vi "2nd_Derivative_Calc_Histogram.vi"(3 "[IN] delta":u16=1 min=1 max=50 step=1, 4 "[IN] Threshold value":u16, 5 "[IN] 1D Sorted Reversed Img":u16[](array[numeric])) -> (1 "[OUT] 2nd Derivative":dbl)   [LabVIEW 2020]
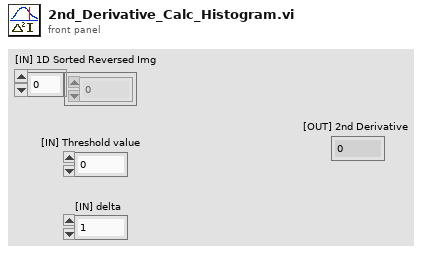
[diagram p1: front panel]
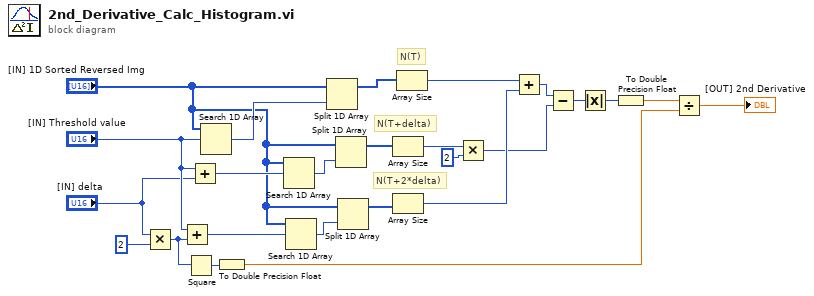
[diagram p0: block diagram]
diagram:
  # "N(T+2*delta)"
  # "N(T+delta)"
  # "N(T)"
  n1 = Multiply(x="[IN] delta", y=u16 2) -> (x*y=w15:u16)
  n2 = Add(x="[IN] Threshold value", y=w15) -> (x+y=w22:u16)
  n3 = Square(x=w15) -> (x^2=w8:u16)
  n4 = Add(x="[IN] Threshold value", y="[IN] delta") -> (x+y=w5:u16)
  n5 = Search 1D Array(1D array="[IN] 1D Sorted Reversed Img", element="[IN] Threshold value") -> (index of element=w24:i32)  [unwired: 1 in]
  n6 = To Double Precision Float(number=w8) -> (double precision float=w6:dbl)
  n7 = Search 1D Array(1D array="[IN] 1D Sorted Reversed Img", element=w5) -> (index of element=w21:i32)  [unwired: 1 in]
  n8 = Search 1D Array(1D array="[IN] 1D Sorted Reversed Img", element=w22) -> (index of element=w19:i32)  [unwired: 1 in]
  n9 = Split 1D Array(array="[IN] 1D Sorted Reversed Img", index=w24) -> (first subarray=w25:u16[])  [unwired: 1 out]
  n10 = Split 1D Array(array="[IN] 1D Sorted Reversed Img", index=w21) -> (first subarray=w20:u16[])  [unwired: 1 out]
  n11 = Split 1D Array(array="[IN] 1D Sorted Reversed Img", index=w19) -> (first subarray=w18:u16[])  [unwired: 1 out]
  n12 = Array Size(array=w20) -> (size(s)=w14:i32)
  n13 = Array Size(array=w18) -> (size(s)=w17:i32)
  n14 = Array Size(array=w25) -> (size(s)=w16:i32)
  n15 = Multiply(x=w14, y=2) -> (x*y=w11:i32)
  n16 = Add(x=w16, y=w17) -> (x+y=w12:i32)
  n17 = Subtract(x=w12, y=w11) -> (x-y=w10:i32)
  n18 = Absolute Value(x=w10) -> (abs(x)=w9:i32)
  n19 = To Double Precision Float(number=w9) -> (double precision float=w7:dbl)
  n20 = Divide(x=w7, y=w6) -> (x/y=→"[OUT] 2nd Derivative":dbl)
